vi "Delete Attributes.vi"(7 "Linked List ID":string, 8 "error in (no error)":errorcluster, 9 "Types":variant[](array[variant]), 10 "Attribute Names":string[](array[string]), 11 "Linked List in":refnum<class "Linked List.lvclass">) -> (0 "error out":errorcluster, 1 "Found?":bool, 3 "Linked List out":refnum<class "Linked List.lvclass">)   [LabVIEW 2020, in "Linked Lists.lvlib" / "Linked List.lvclass"]
uses:
  <vilib>/gpm_packages/@cs/linked-list/Source/Linked List/Linked List/Linked List.lvclass
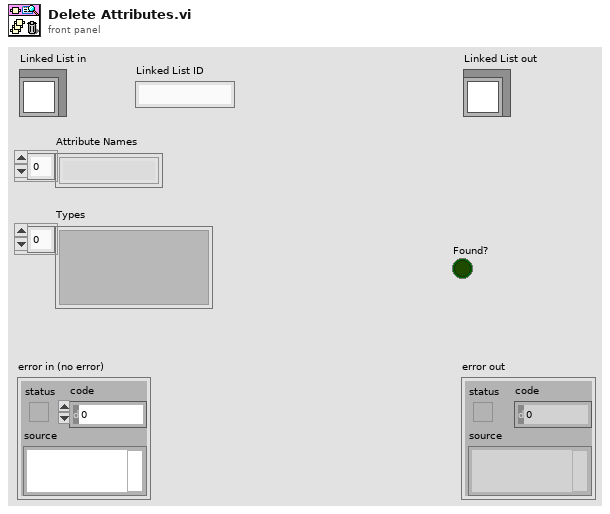
[diagram p1: front panel]
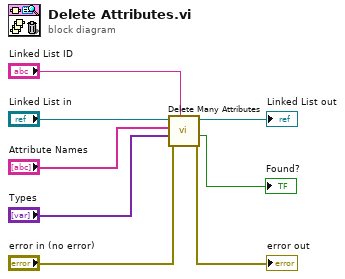
[diagram p0: block diagram]
diagram:
  n1 = call <vilib>:"Delete Many Attributes.vi"("Unique ID"="Linked List ID", "error in (no error)"="error in (no error)", "Types"="Types", "Attribute Names"="Attribute Names", "Linked List in"="Linked List in") -> ("error out"=→"error out":errorcluster, "Found?"=→"Found?":bool, "Linked List out"=→"Linked List out":refnum<class "Linked List.lvclass">)  [unwired: 4 in]
